vi "(SubVI) Trigger a Sine Wave Configuration.vi"(4 "error in (no error)":errorcluster, 6 "Axis  (Enum)":enum16{"x", "y", "z"}(ring)) -> (0 "error out":errorcluster)   [LabVIEW 2014]
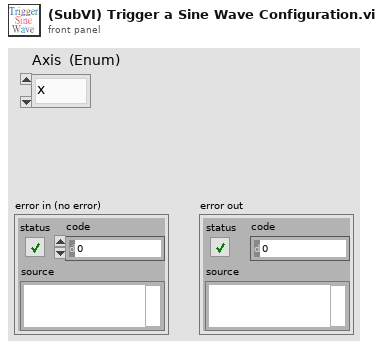
[diagram p1: front panel]
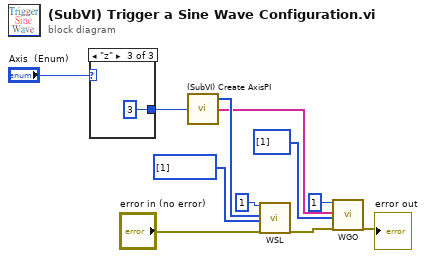
[diagram p0: block diagram]
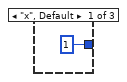
[diagram p2: hidden frame]
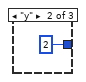
[diagram p3: hidden frame]
diagram:
  n1 = case shown="\"z\"" "Axis  (Enum)" {
    tunnel: [1 2 3] -> w1
    frame "x", Default {
    }
    frame "y" {
    }
    frame "z" {
    }
  }
  n2 = call "(SubVI) Create AxisPI.vi"("axis"=w1) -> ("Axis String Array"=w3:string[], "Axis Array"=w4:i32[])  [unwired: 2 in, 1 out]
  n3 = call "WSL.vi"("System no."=1, "Generator ID"=w4, "WaveTableID"=i32[] [1], "error in"="error in (no error)") -> ("error out"=w7:errorcluster)  [unwired: 15 out]
  n4 = call "WGO.vi"("System no."=1, "Affected axes"=w3, "WGO Parameter"=i32[] [1], "error in"=w7) -> ("error out"=→"error out":errorcluster)  [unwired: 15 out]
